vi "Read Alias.vi"(11 "Power Supply in":refnum<class "Power Supply.lvclass">) -> (2 "Alias":string, 3 "Power Supply out":refnum<class "Power Supply.lvclass">)   [LabVIEW 2020, in "Power Supply.lvclass"]
uses:
  Power Supply.lvclass
  Power Supply.lvclass/Power Supply.ctl
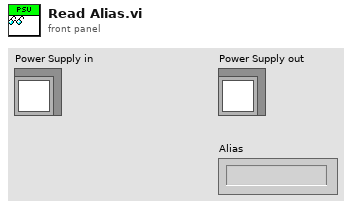
[diagram p1: front panel]
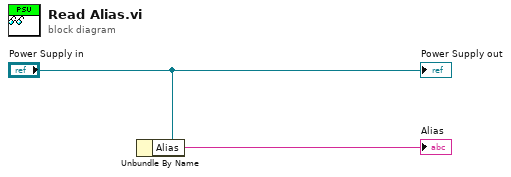
[diagram p0: block diagram]
diagram:
  n1 = Unbundle By Name("Power Supply in") -> ("Alias"=→"Alias":string)
  "Power Supply out" <- "Power Supply in"
